vi "Add Array.vi"(6 "Parent (None)":string[](array[string]), 8 "error in (no error)":errorcluster, 10 "Name":string, 11 "TemplateLocals in":refnum<class "Value Tree.lvclass">) -> (0 "error out":errorcluster, 3 "TemplateLocals out":refnum<class "Value Tree.lvclass">, 4 "Hierarchy":string[](array[string]))   [LabVIEW 2020, in "HTTP Server.lvlib" / "Value Tree.lvclass"]
uses:
  Value Tree.lvclass
  Local Type.ctl
  Value Tree.lvclass/Value Tree.ctl
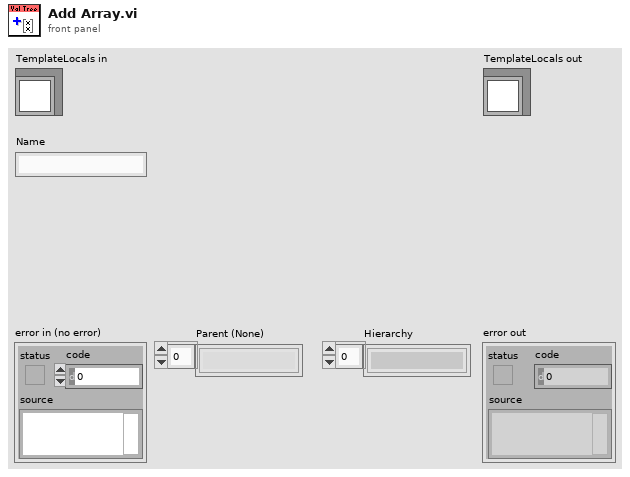
[diagram p1: front panel]
types:
  T1 = typedef "HTTP Server.lvlib/Value Tree.lvclass/Local Type.ctl" = enum16{"Scalar", "Object", "Array"}
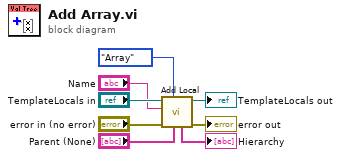
[diagram p0: block diagram]
diagram:
  n1 = call "Add Local.vi"("Parent"="Parent (None)", "Type"=Local_Type."Array", "error in (no error)"="error in (no error)", "Name"="Name", "TemplateLocals in"="TemplateLocals in") -> ("error out"=→"error out":errorcluster, "TemplateLocals out"=→"TemplateLocals out":refnum<class "Value Tree.lvclass">, "Hierarchy"=→"Hierarchy":string[])  [unwired: 4 in]
